vi "纳清电导率电极校准.vi"() -> ()   [LabVIEW 2016, in "斯坦道多参数.lvlib"]
uses:
  <vilib>/Utility/miscctls.llb/LVPointTypeDef.ctl
  <vilib>/Analysis/NI_AALBase.lvlib
panel:
  out "滤波设定":sgl
  out "第二点信号值":dbl
  out "第一点信号值":dbl
  out "盐度":dbl caption="盐度测量值" format="%#.2f"
  out "当前量程":u16
  out "报警信息":string
  out "通讯状态":string
  out "第二点校准值":dbl
  out "第一点校准值":dbl
  in  "校准停止":bool
  in  "校准启动":bool
  in  "校准模式":u16(ring) items=["单点校准"]
  out "最小值":sgl format="%#.2f"
  out "最大值":sgl format="%#.2f"
  out "波形图表":dbl(graph) caption="历史曲线"
  out "mean":dbl caption="均值" format="%#.2f"
  out "standard deviation":dbl caption="标准差" format="%#.2f"
  out "变异系数":dbl format="%#.6f"
  out "测量值":sgl format="%#.2f"
  out "提示":string
  out "标液1":sgl
  out "原始光强数值":sgl caption="信号值" format="%#.6f"
  out "温度":dbl format="%#.2f"
  # "电导率电极设定"
  # "℃"
  # "μS/cm"
  # "ppt"
  # "电阻"
  # "请选择校准模式:"
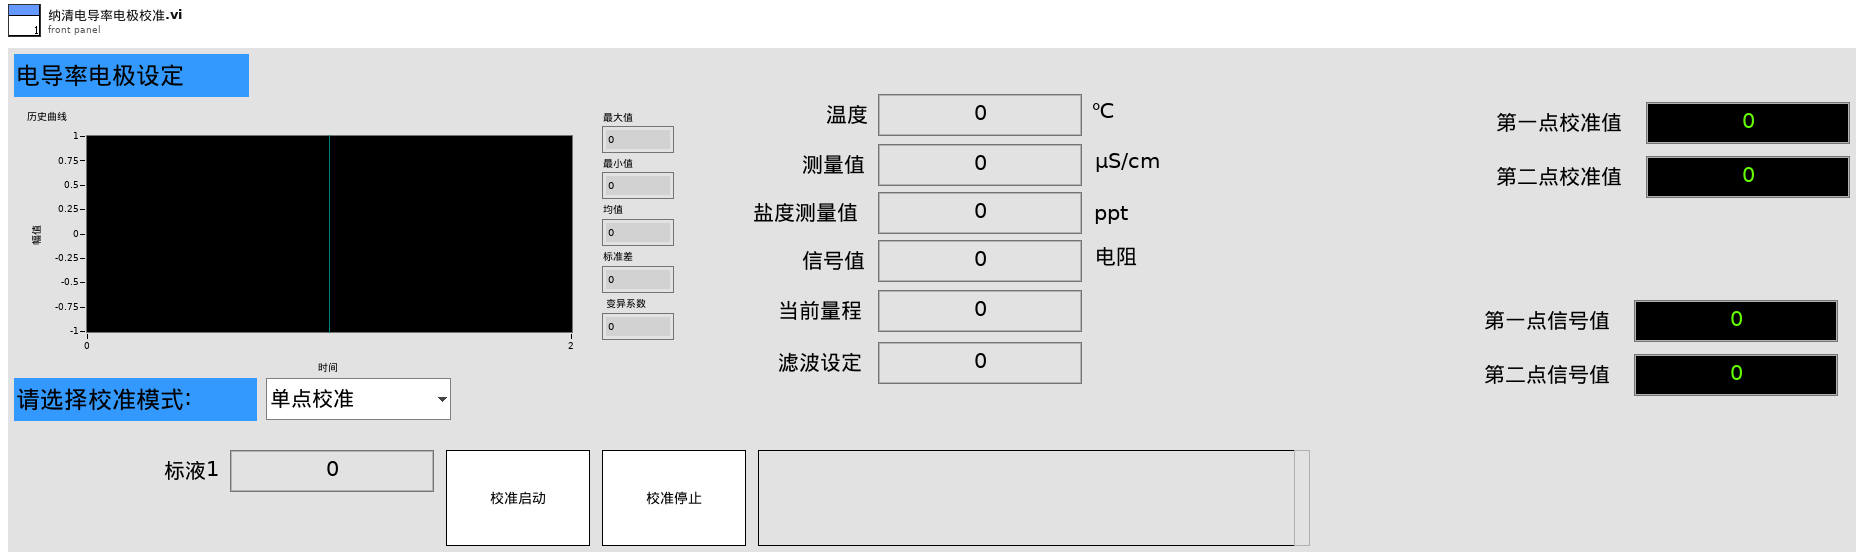
[diagram p1: front panel]
types:
  T1 = enum16{"pH", "DO", "Cond", "Turb", "ORP", "叶绿素a", "藻密度"}
  T2 = typedef "LVPointTypeDef.ctl" = cluster{"Horizontal":i16, "Vertical":i16}
  T3 = cluster{"报警码":u16, "电导率数据（uS/cm）":sgl, "0x0003 NC":sgl, "温度数据":sgl, "电导率原始信号电阻":sgl, "当前量程":u16, "温度补偿系数":sgl, "0X0009_NC":string, "产品名称":string, "序列号":string, "硬件版本":string, "软件版本":string, "通讯地址":u16, "波特率":u16, "设备类型":u16, "0X0026_NC":string, "第一点原始数据":sgl, "第一点校准数据":sgl, "0X0035_NC":sgl, "0X0037_NC":sgl, "探头校准命令":u16, "温度校准参数":sgl, "温度校准命令":u16}
  T4 = cluster{"温度测量值":sgl, "测量值":sgl, "温度偏移修正值":sgl, "信号值":sgl}
  T5 = cluster{"pH":u32, "DO":u32, "Cond":u32, "Turb":u32, "叶绿素a":u32, "藻密度":u32, "ORP":u32}
  T6 = enum8{"Enabled", "Disabled", "Disabled and Grayed Out"}
  T7 = cluster{"ph":bool, "DO":bool, "Cond":bool, "Turb":bool, "叶绿素a":bool, "藻密度":bool, "ORP":bool}
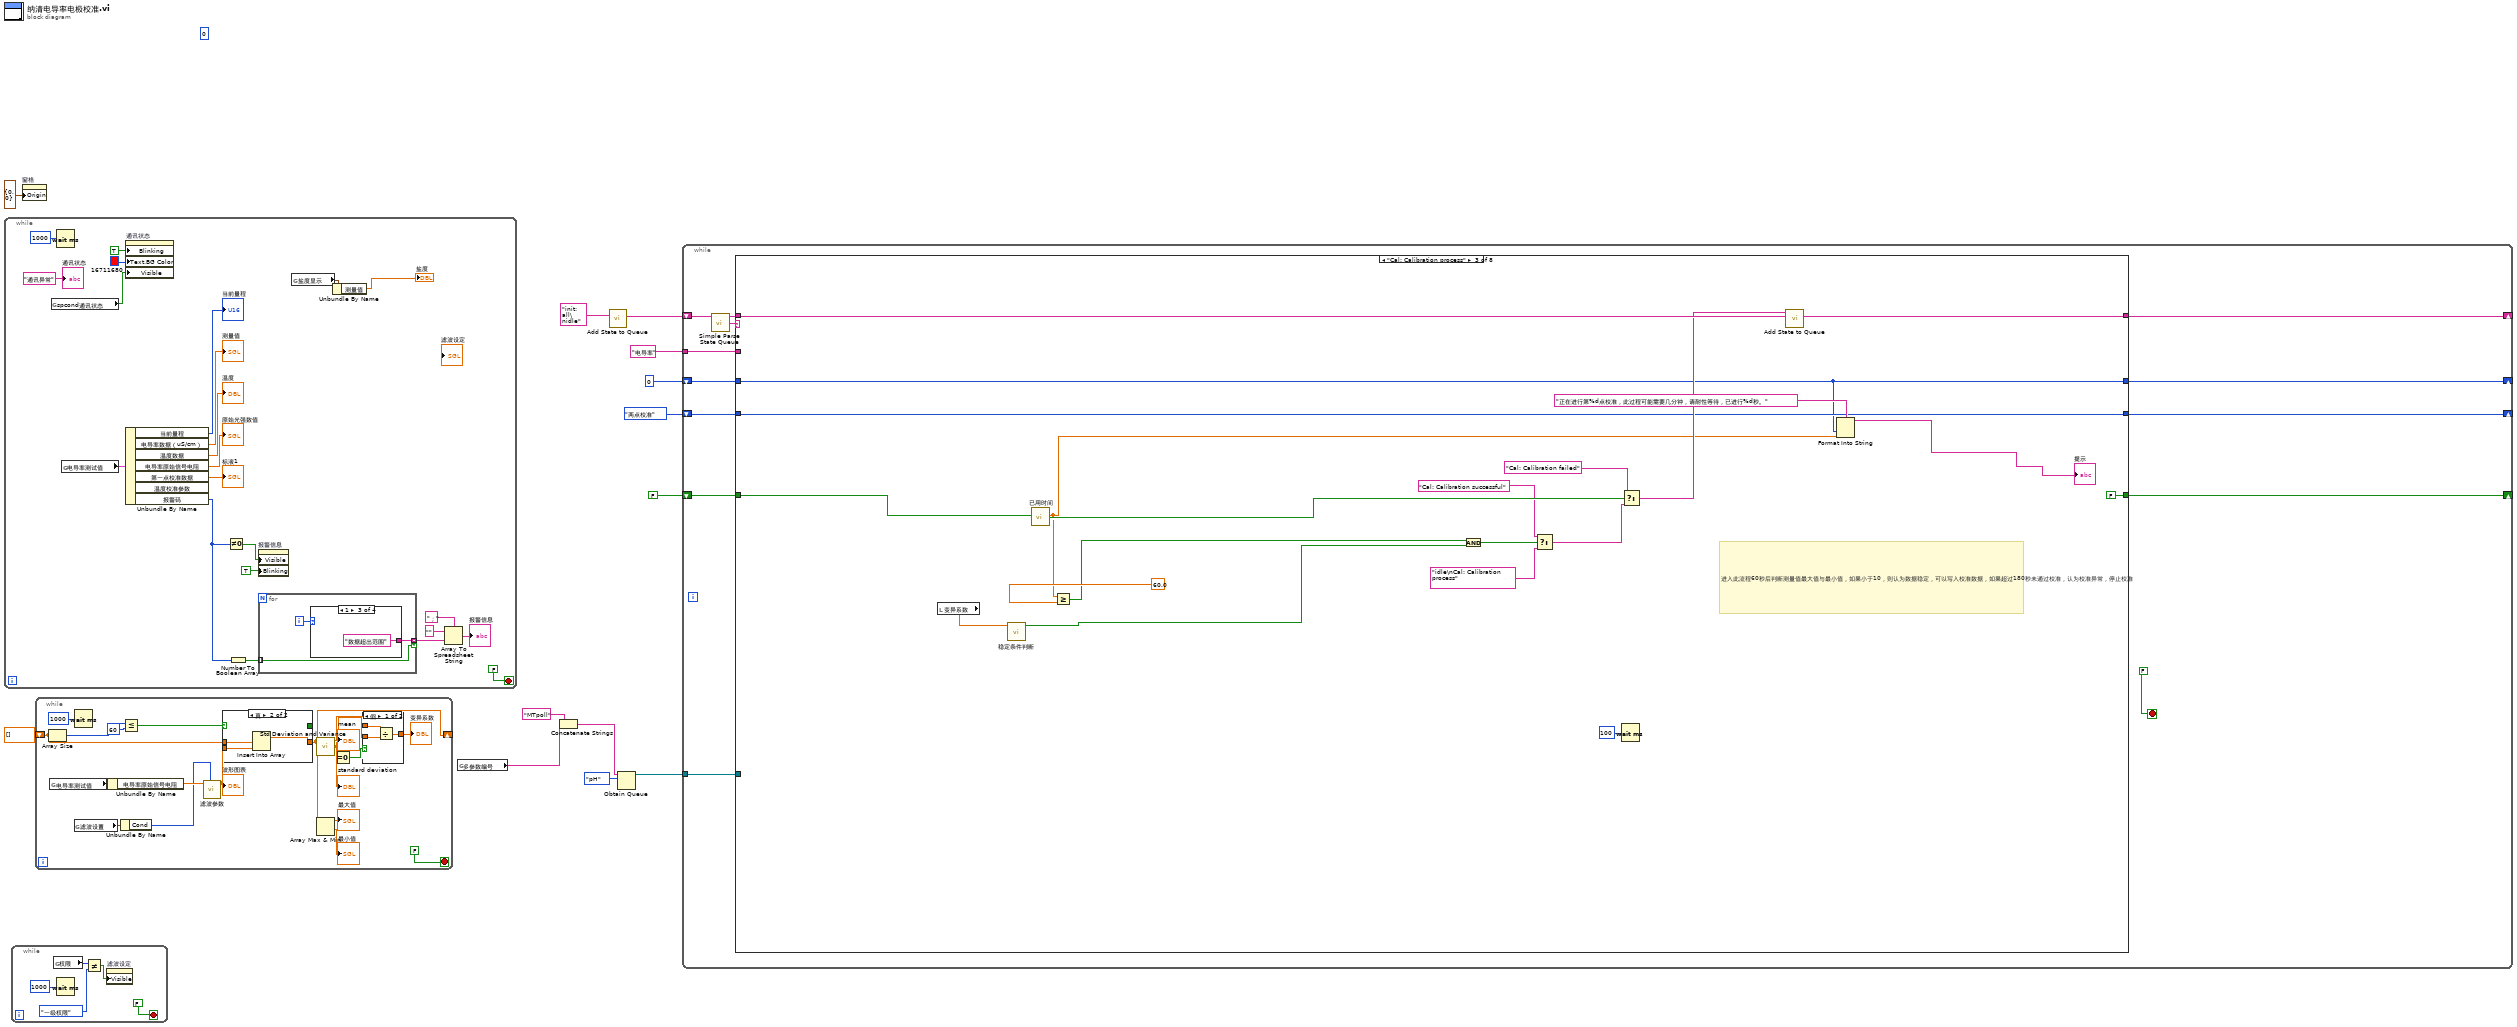
[diagram p0: block diagram]
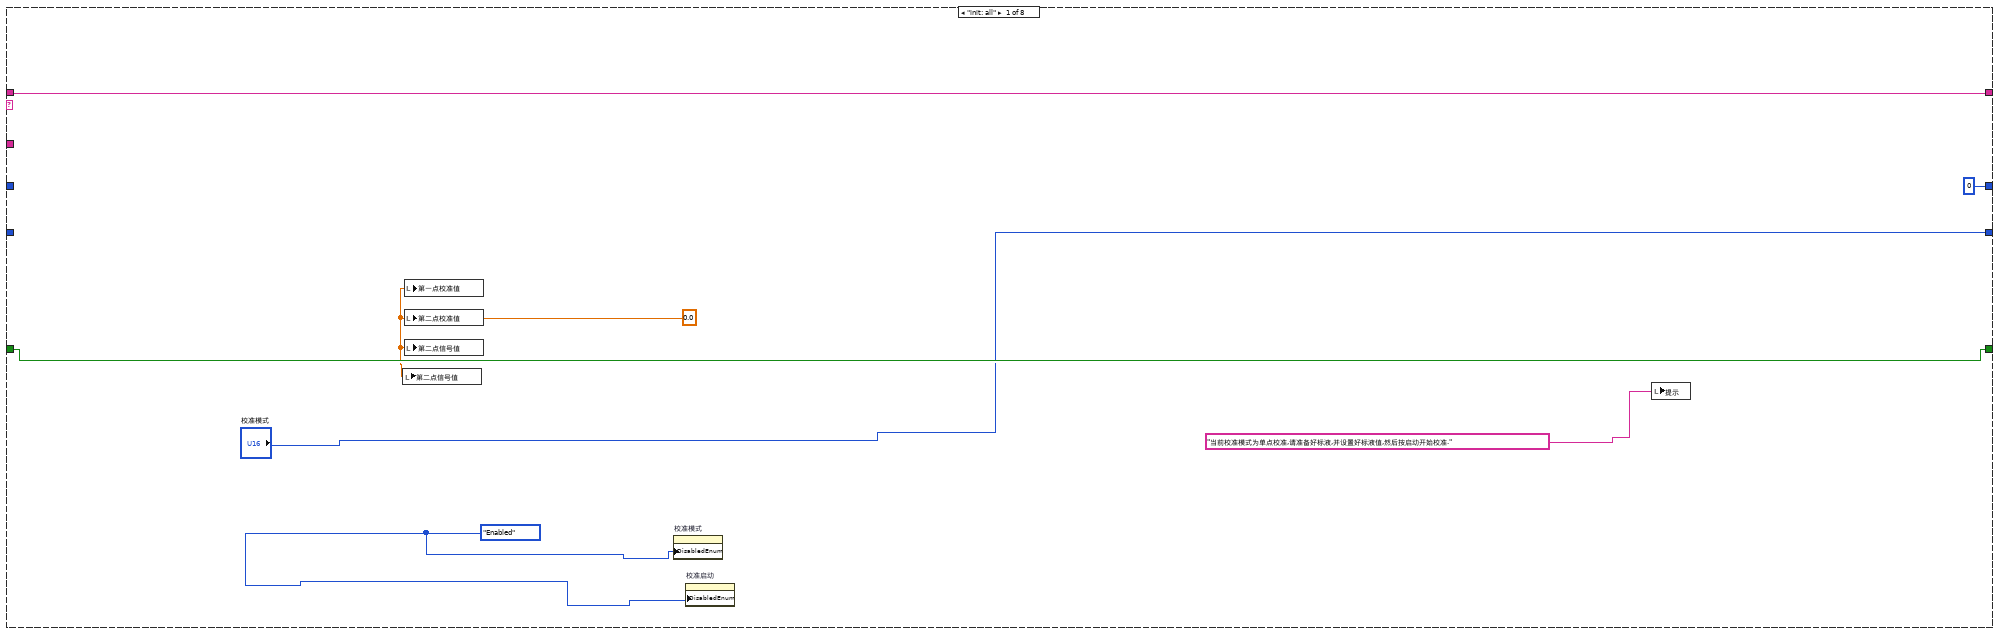
[diagram p2: hidden frame]
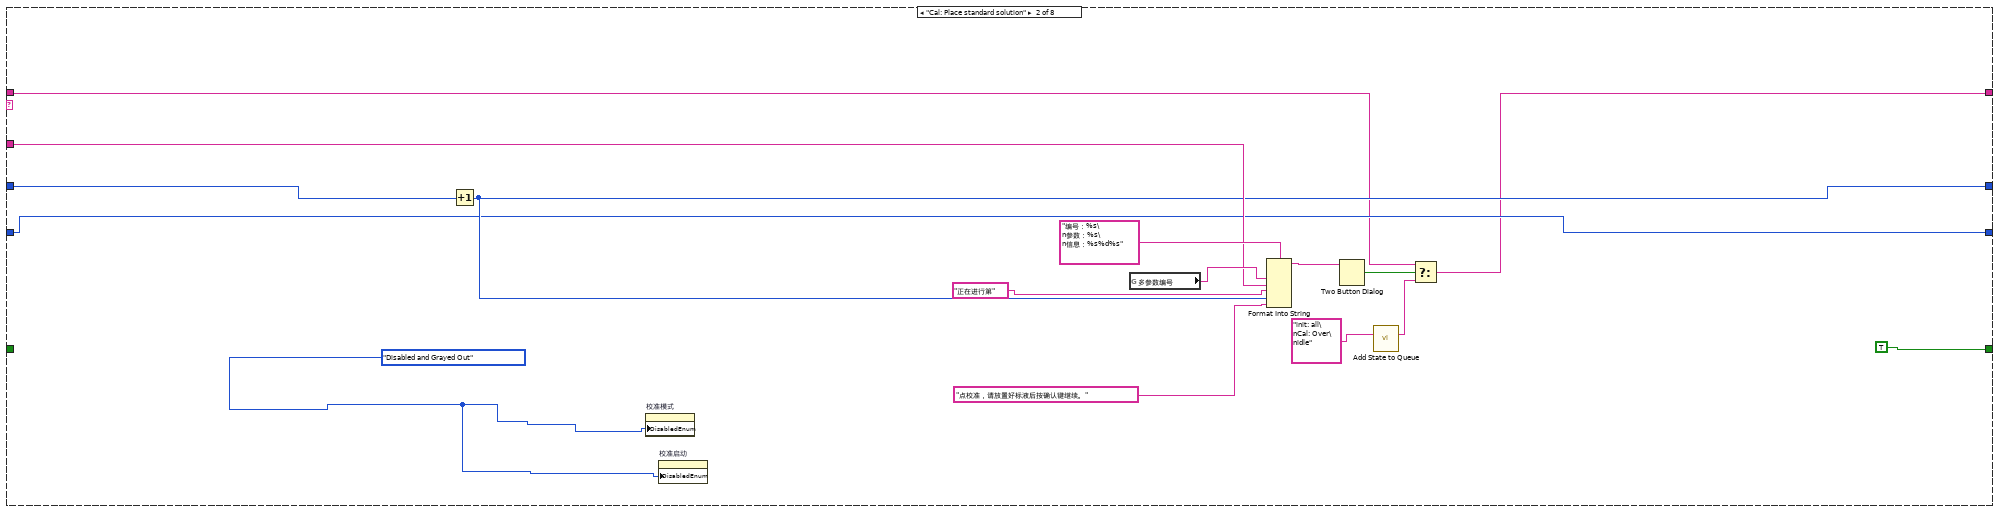
[diagram p3: hidden frame]
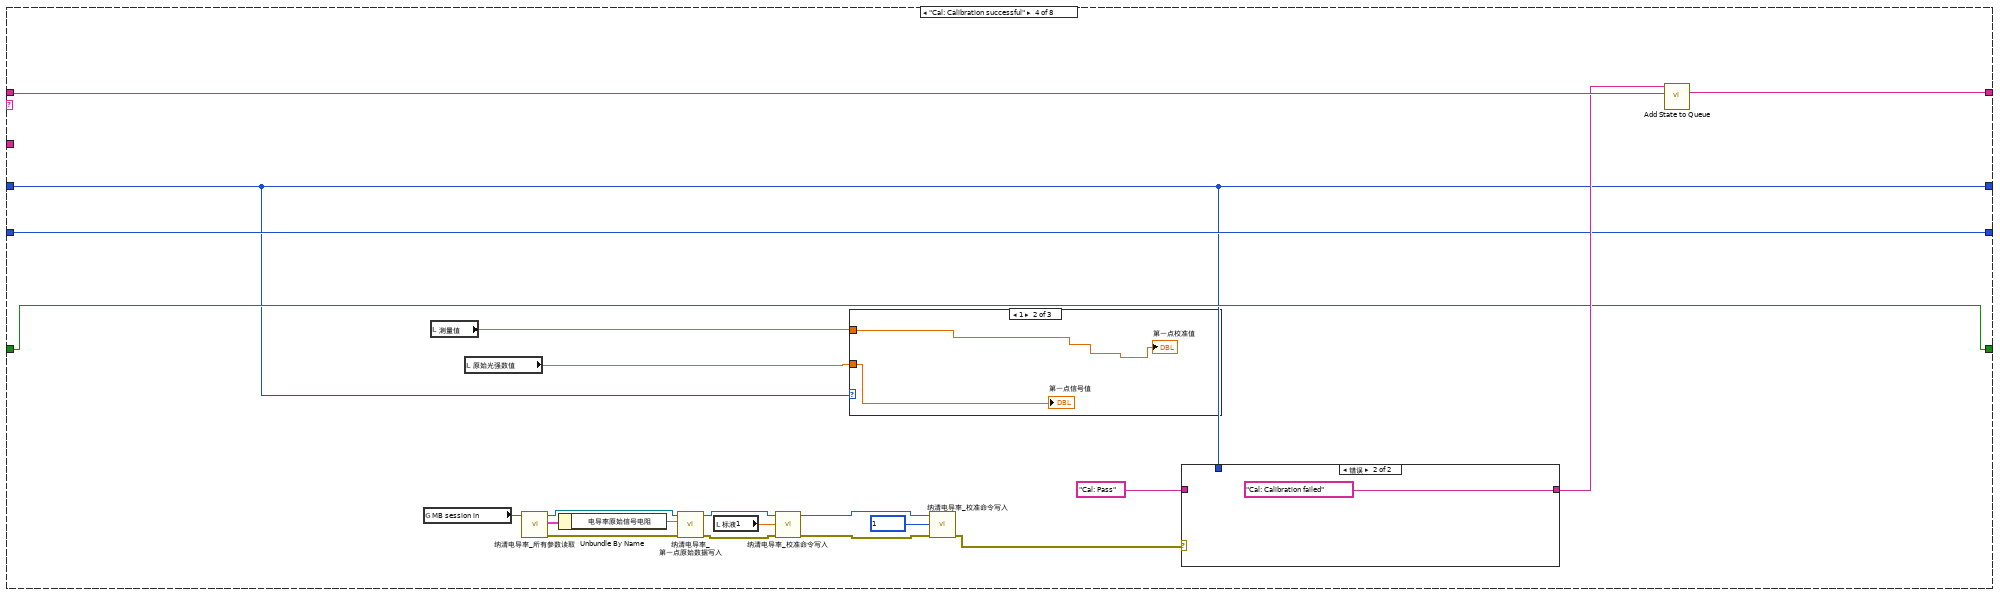
[diagram p4: hidden frame]
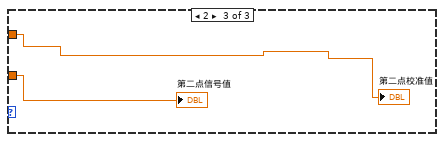
[diagram p6: hidden frame]
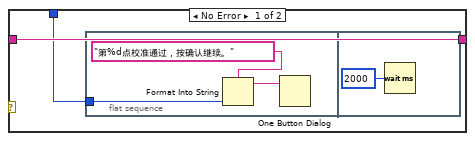
[diagram p7: hidden frame]
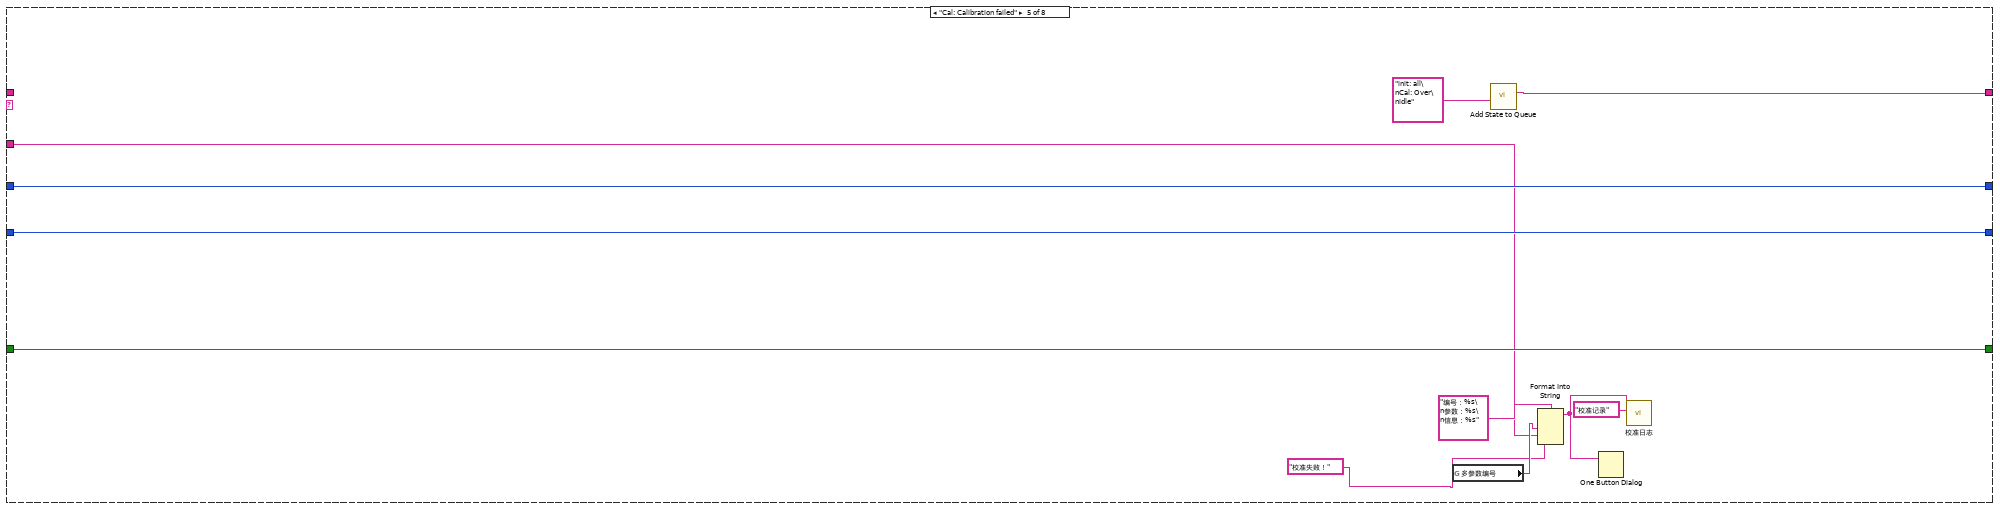
[diagram p8: hidden frame]
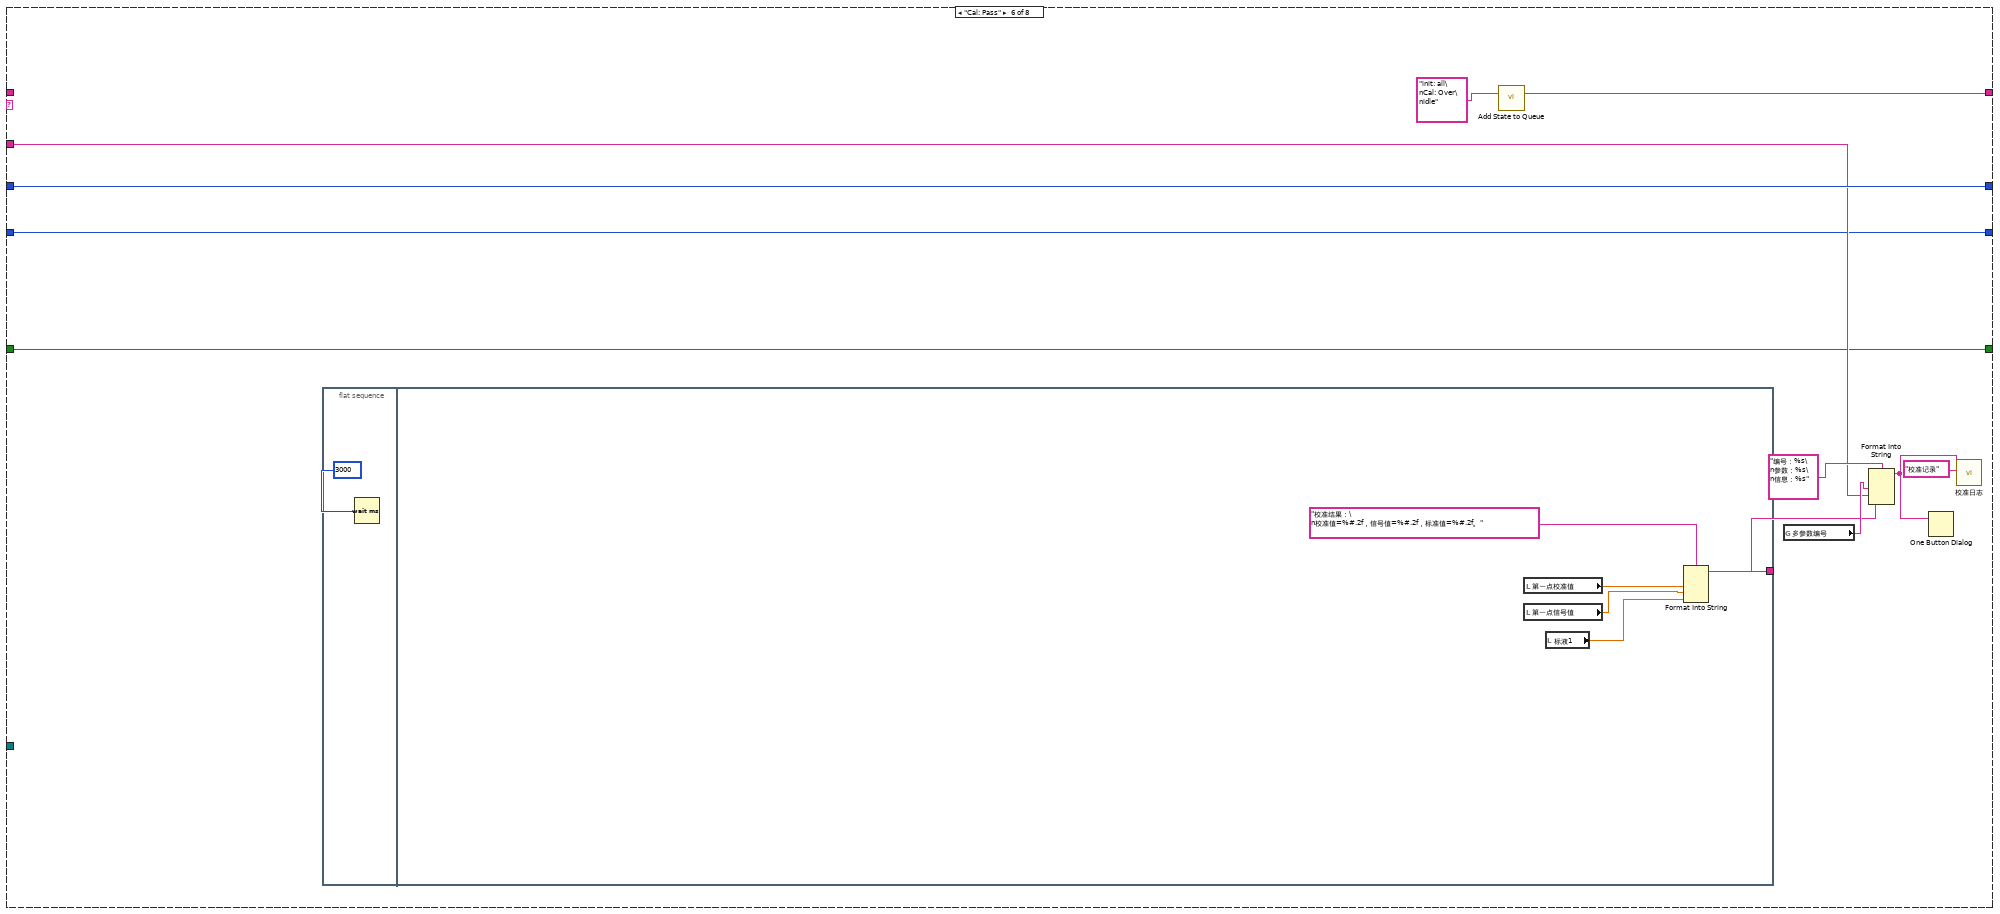
[diagram p9: hidden frame]
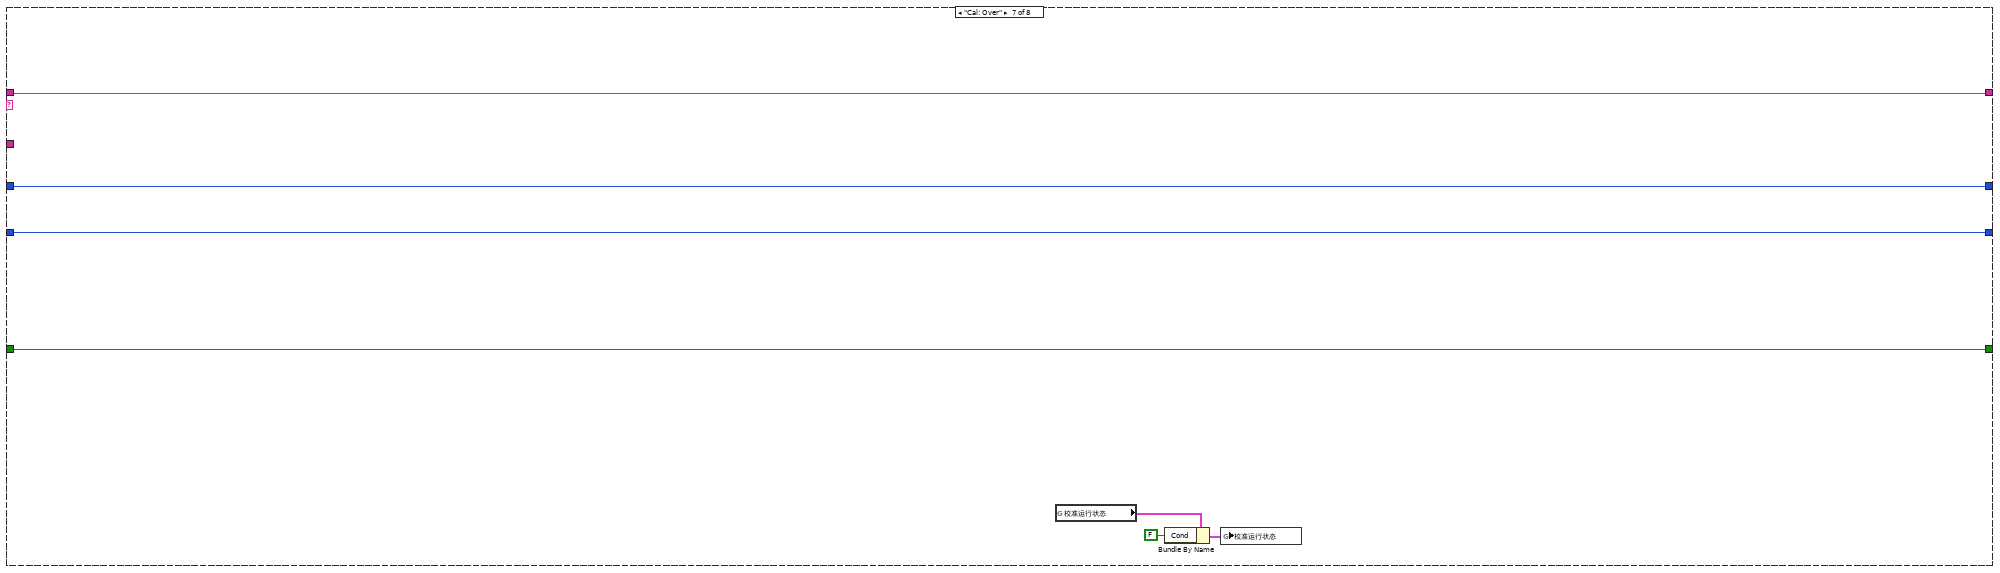
[diagram p10: hidden frame]
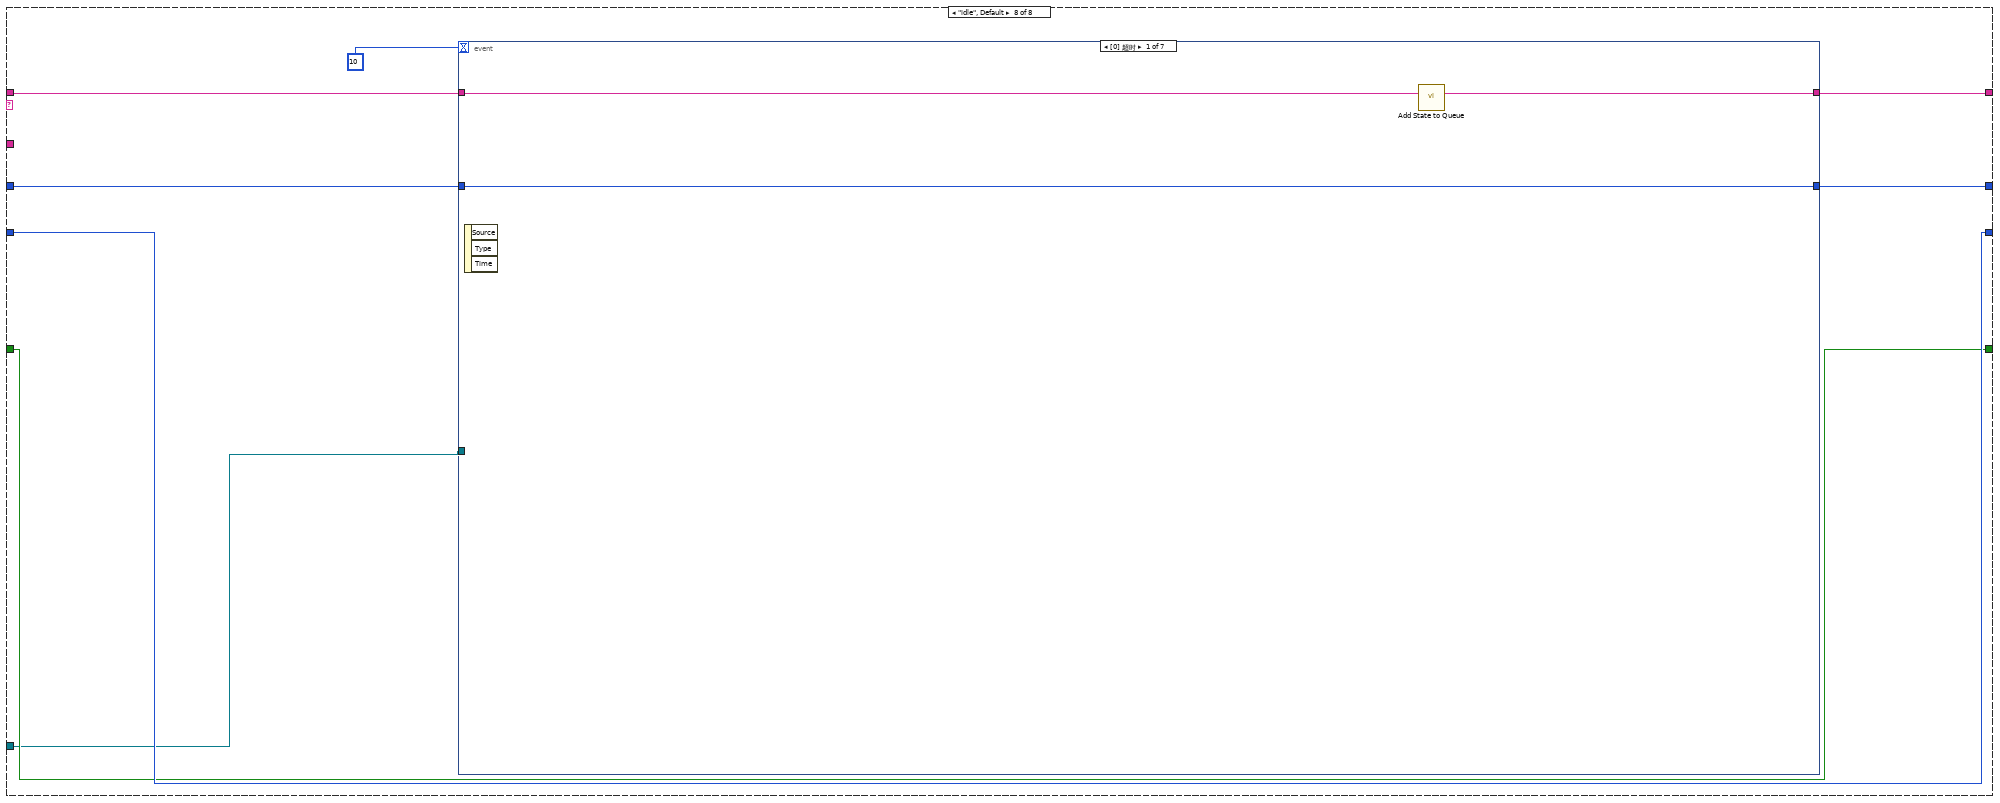
[diagram p11: hidden frame]
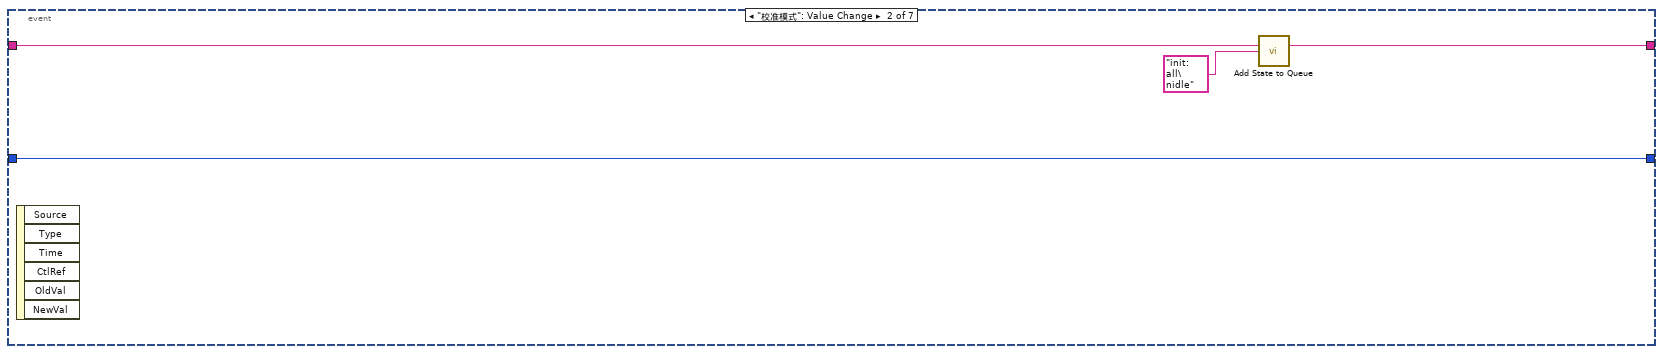
[diagram p12: hidden frame]
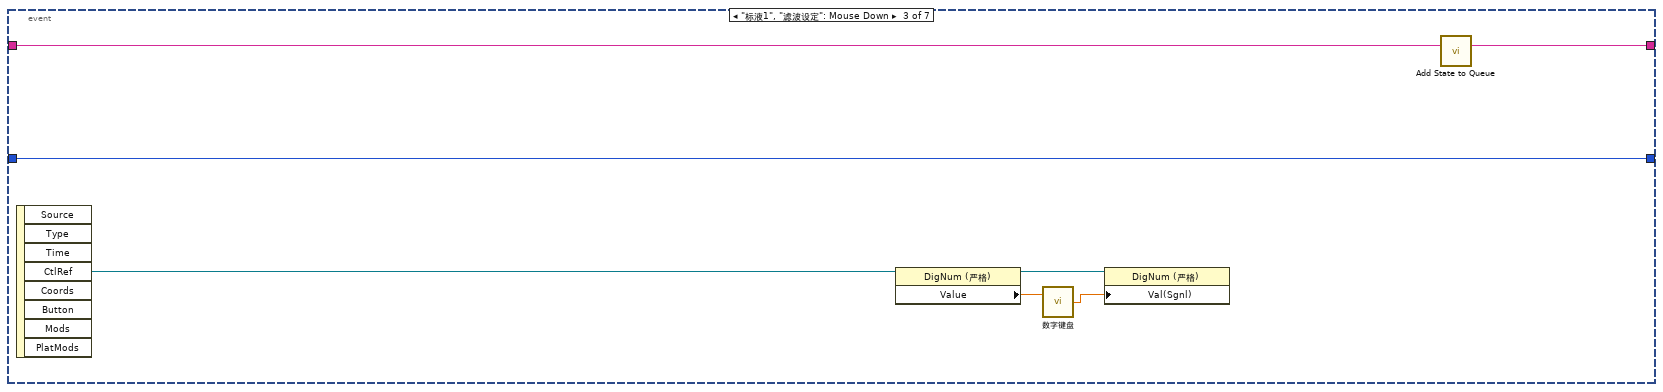
[diagram p13: hidden frame]
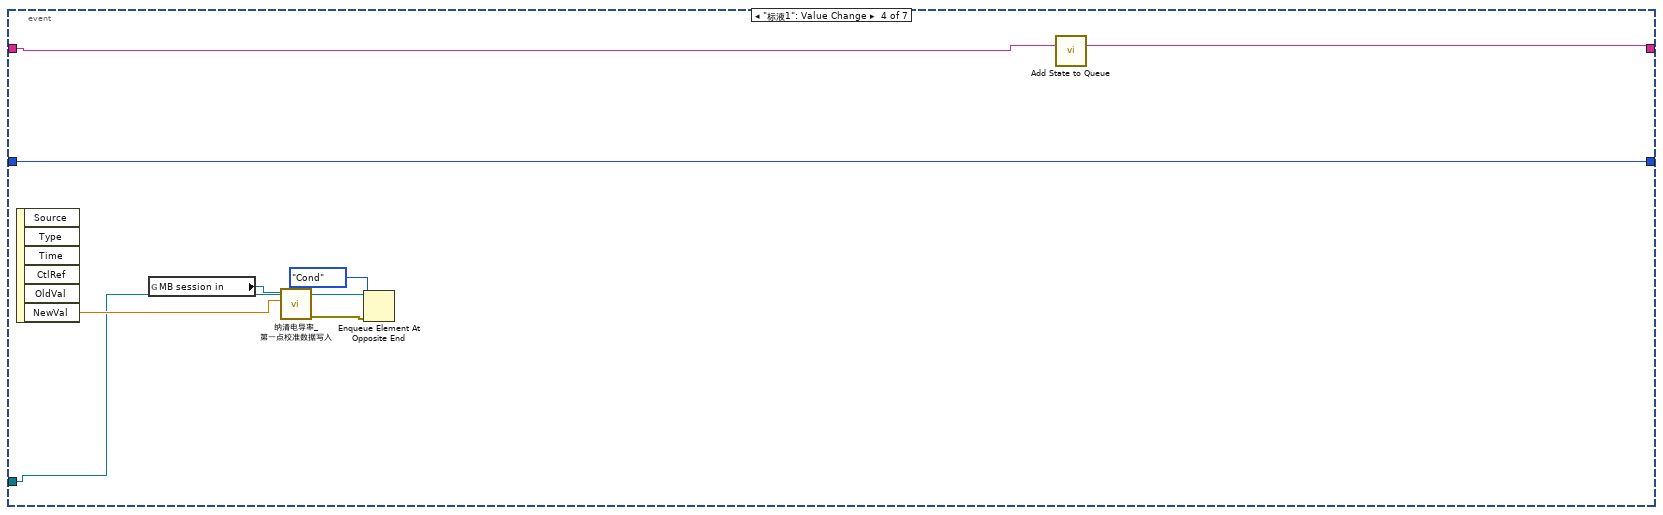
[diagram p14: hidden frame]
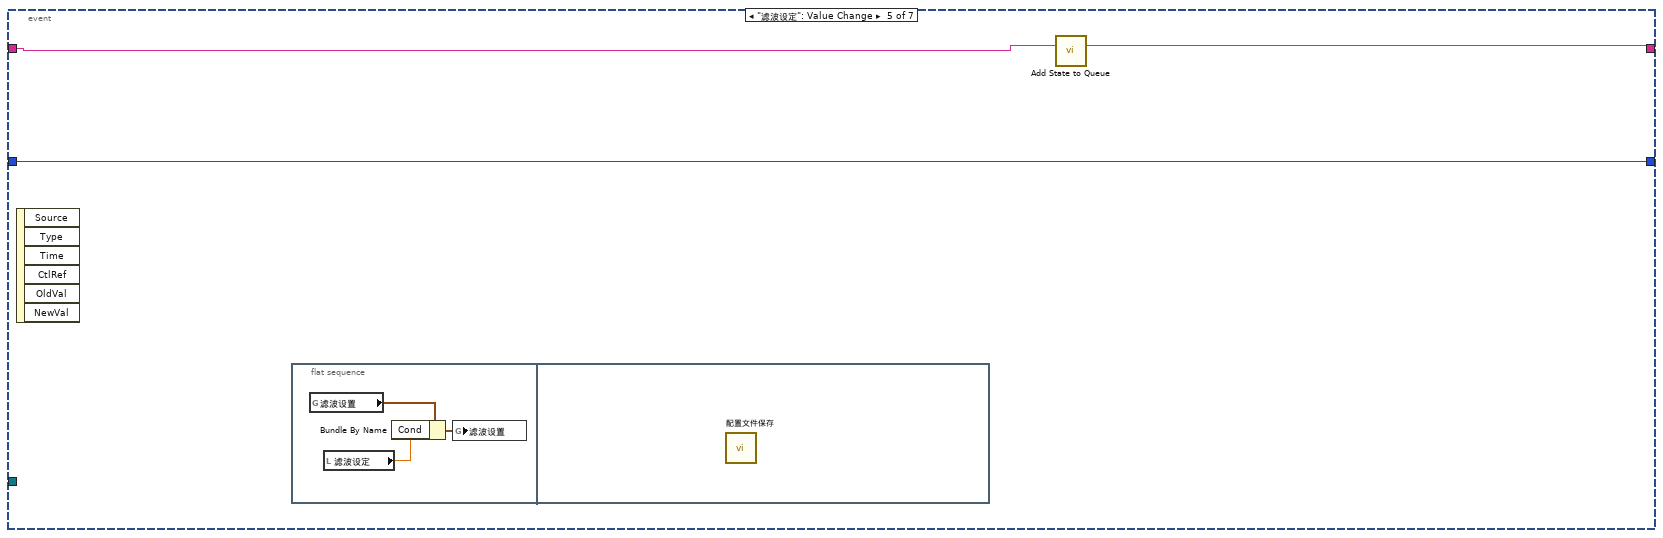
[diagram p15: hidden frame]
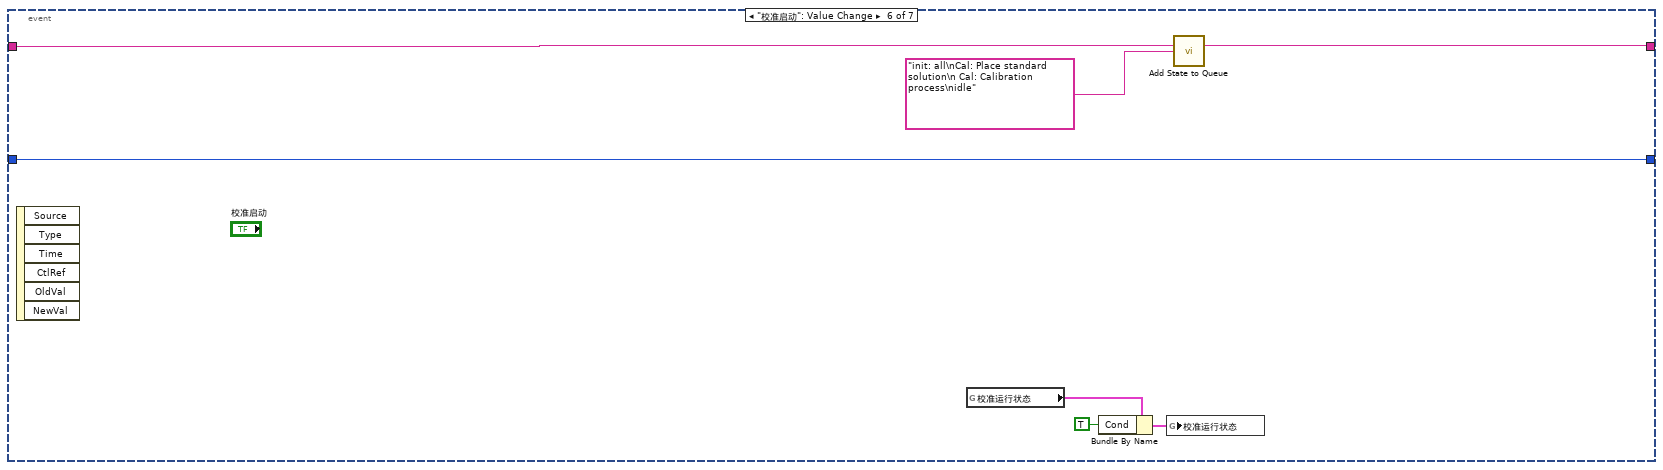
[diagram p16: hidden frame]
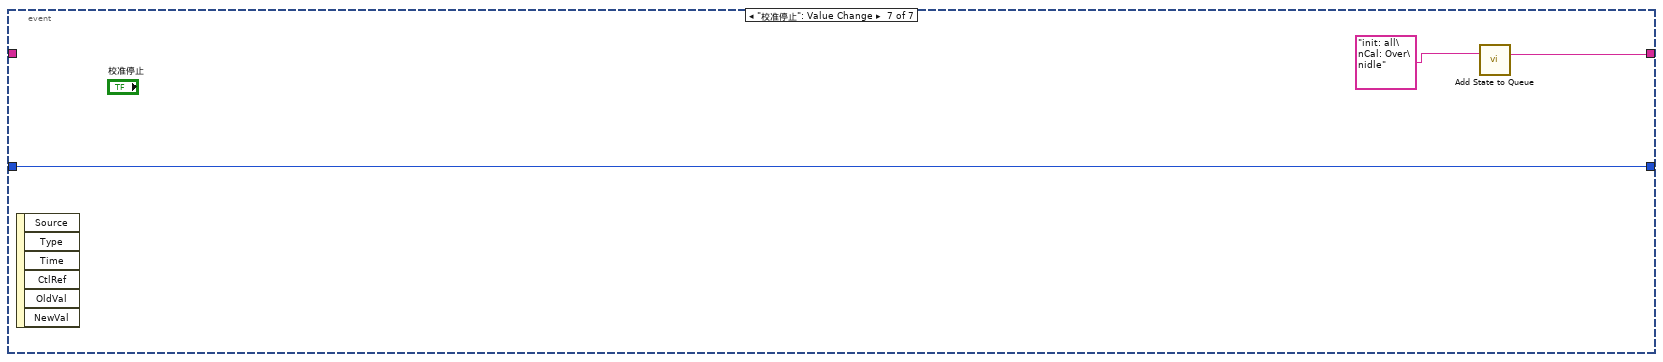
[diagram p17: hidden frame]
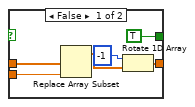
[diagram p19: hidden frame]
diagram:
  (unwired) 0
  n1 = while {
    stop <- FALSE stop-if-true
    n2 = global read "多参数全局变量.vi" "spcond通讯状态"() -> (w25:bool)
    n3 = Wait (ms)(milliseconds to wait=u32 1000 ("等待时间（毫秒）")) -> ()  [unwired: 1 out]
    n4 = global read "纳清过程全局变量.vi" "电导率测试值"() -> (w33:T3)
    n5 = property on="通讯状态" class="Str"("Blinking"=TRUE ("闪烁"), "Text.BG Color"=u32 16711680, "Visible"=w25) -> ()  [unwired: 2 in, 2 out]
    n6 = Unbundle By Name(w33) -> ("当前量程"=→"当前量程":u16, "电导率数据（uS/cm）"=→"测量值":sgl, "温度数据"=→"温度":sgl, "电导率原始信号电阻"=→"原始光强数值":sgl, "第一点校准数据"=→"标液1":sgl, "报警码"=w19:u16)  [unwired: 1 out]
    n7 = Not Equal To 0?(x=w19) -> (x != 0?=w18:bool)
    n8 = Number To Boolean Array(number=w19) -> (Boolean array=w24:bool[])
    n9 = property on="报警信息" class="Str"("Visible"=w18, "Blinking"=TRUE ("闪烁")) -> ()  [unwired: 2 in, 2 out]
    n10 = for {
      tunnel: w24 -> [w36] mode=indexing
      tunnel: [w37] -> w23 mode=indexing if=w36
      i -> [w38]
      n11 = case shown="1" w38 {
        tunnel: [_ "温度超出范围" "数据超出范围" "温度传感器故障"] -> w37
        frame Default {
        }
        frame 0 {
        }
        frame 1 {
        }
        frame 8 {
        }
      }
    }
    n12 = global read "多参数全局变量.vi" "盐度显示"() -> (w14:T4)
    n13 = Unbundle By Name(w14) -> ("测量值"=→"盐度":sgl)
    n14 = Array To Spreadsheet String(delimiter (Tab)="；" ("分隔符(Tab)"), array=w23, 3:"" ("格式字符串")) -> (spreadsheet string=→"报警信息":string)
    "通讯状态" <- "通讯异常" ("当前串口")
  }
  n15 = while {
    stop <- FALSE stop-if-true
    n16 = global read "多参数全局变量.vi" "权限"() -> (w45:enum16{"一级权限", "二级权限", "三级权限"})
    n17 = Wait (ms)(milliseconds to wait=u32 1000 ("等待时间（毫秒）")) -> ()  [unwired: 1 out]
    n18 = Not Equal?(x=w45, y=enum16{"一级权限", "二级权限", "三级权限"}."一级权限") -> (x != y?=w42:bool)
    n19 = property on="滤波设定" class="DigNum (严格)"("Visible"=w42) -> ()  [unwired: 2 in, 2 out]
  }
  n20 = property on="窗格" class="Pane"("Origin"=T2 {"Horizontal"=0, "Vertical"=0} ("原点")) -> ()  [unwired: 2 in, 2 out]
  n21 = while {
    shift-right: [w54] -> _
    shift-left: sgl[] [] -> [w60]
    stop <- FALSE stop-if-true
    n22 = Array Size(array=w60) -> (size(s)=w62:i32)
    n23 = global read "纳清过程全局变量.vi" "电导率测试值"() -> (w51:T3)
    n24 = global read "断电保存变量.vi" "滤波设置"() -> (w48:T5)
    n25 = Wait (ms)(milliseconds to wait=u32 1000 ("等待时间（毫秒）")) -> ()  [unwired: 1 out]
    n26 = Unbundle By Name(w51) -> ("电导率原始信号电阻"=w50:sgl)
    n27 = Unbundle By Name(w48) -> ("Cond"=w47:u32)
    n28 = Less Or Equal?(x=w62, y=60) -> (x <= y?=w61:bool)
    n29 = call "滤波参数.vi"("滤波次数"=w47, "x"=w50) -> ("mode"=w49:dbl)  [unwired: 9 in]
    "波形图表" <- w49
    n30 = case shown="真" w61 {
      tunnel: w60 -> [w73 w76]
      tunnel: w49 -> [w71 w75]
      tunnel: [w69 w74] -> w54
      tunnel: [TRUE _] -> _
      frame False {
        n31 = Replace Array Subset(array=w73, new element=w71) -> (w72:sgl[])  [unwired: 1 in]
        n32 = Rotate 1D Array(1:w72, 2:-1 ("n")) -> (0:w69:sgl[])
      }
      frame True {
        n33 = Insert Into Array(array=w76, new element=w75) -> (w74:sgl[])  [unwired: 1 in]
      }
    }
    n34 = call <vilib>:"Std Deviation and Variance.vi"("X"=w54) -> ("mean"=w58:dbl, "standard deviation"=w57:dbl)  [unwired: 1 in, 1 out]
    "mean" <- w58
    "standard deviation" <- w57
    n35 = Array Max & Min(array=w54) -> (max value=→"最大值":sgl, min value=→"最小值":sgl)  [unwired: 2 out]
    n36 = Equal To 0?(x=w58) -> (x = 0?=w59:bool)
    n37 = case shown="假" w59 {
      tunnel: w57 -> [w67 _]
      tunnel: [w66 _] -> w56
      tunnel: w58 -> [w65 _]
      frame False {
        n38 = Divide(x=w67, y=w65) -> (x/y=w66:dbl)
      }
      frame True {
      }
    }
    "变异系数" <- w56
  }
  n39 = global read "多参数全局变量.vi" "多参数编号"() -> (w2:string)
  n40 = Concatenate Strings("MTpoll" ("名称（未命名）"), w2) -> (w4:string)
  n41 = call "Add State to Queue.vi"("State(s) In (\"\")"="init: all\nidle" ("State(s) In (\"\")")) -> ("States Out"=w10:string)  [unwired: 14 in]
  n42 = Obtain Queue(name (unnamed)=w4, element data type=T1."pH" ("枚举")) -> (queue out=w1:refnum<queue>)  [unwired: 3 in, 2 out]
  n43 = while {
    shift-right: [w85] -> _
    shift-left: w10 -> [w89]
    shift-right: [w82] -> _
    shift-left: 0 -> [w84]
    tunnel: "电导率" ("State(s) In (\"\")") -> [w83]
    shift-right: [w80] -> _
    shift-left: enum16{"两点校准", "单点校准"}."两点校准" ("校准模式") -> [w81]
    shift-right: [w78] -> _
    shift-left: FALSE -> [w79]
    tunnel: w1 -> [w77]
    stop <- FALSE stop-if-true
    n44 = call "Simple Parse State Queue.vi"("State Queue"=w89) -> ("Remain States"=w86:string, "Next State"=w87:string)  [unwired: 13 in]
    n45 = case shown="\"Cal: Calibration process\"" w87 {
      tunnel: w86 -> [w96 w99 w132 w153 _ _ w200 w208]
      tunnel: [w96 w98 w131 w152 w173 w177 w200 w207] -> w85
      tunnel: w84 -> [_ w108 w117 w135 w176 w187 w199 w205]
      tunnel: w83 -> [_ w109 _ _ w166 w183 _ _]
      tunnel: [0 w106 w117 w135 w176 w187 w199 w206] -> w82
      tunnel: w81 -> [_ w105 w118 w147 w175 w179 w198 w204]
      tunnel: ["校准模式" w105 w118 w147 w175 w179 w198 w204] -> w80
      tunnel: w79 -> [w93 _ w120 w148 w174 w182 w197 w202]
      tunnel: [w93 TRUE FALSE w148 w174 w182 w197 w202] -> w78
      tunnel: w77 -> [_ _ _ _ _ _ _ w201]
      frame "init: all" {
        w90 = T6."Enabled" ("禁用")
        w92 = 0.0 ("第一点校准值")
        n46 = local write "第二点信号值"(w92) -> ()
        n47 = local write "第一点校准值"(w92) -> ()
        n48 = local write "第二点校准值"(w92) -> ()
        n49 = local write "第二点信号值"(w92) -> ()
        n50 = property on="校准模式" class="Ring (严格)"("DisabledEnum"=w90) -> ()  [unwired: 2 in, 2 out]
        n51 = property on="校准启动" class="Bool"("DisabledEnum"=w90) -> ()  [unwired: 2 in, 2 out]
        n52 = local write "提示"("当前校准模式为单点校准,请准备好标液,并设置好标液值,然后按启动开始校准." ("提示")) -> ()
      }
      frame "Cal: Place standard solution" {
        w97 = T6."Disabled and Grayed Out" ("禁用")
        n53 = Increment(x=w108) -> (x+1=w106:i32)
        n54 = property on="校准模式" class="Ring (严格)"("DisabledEnum"=w97) -> ()  [unwired: 2 in, 2 out]
        n55 = property on="校准启动" class="Bool"("DisabledEnum"=w97) -> ()  [unwired: 2 in, 2 out]
        n56 = global read "多参数全局变量.vi" "多参数编号"() -> (w111:string)
        n57 = Format Into String(format string="编号：%s\n参数：%s\n信息：%s%d%s" ("格式字符串"), w111, w109, "正在进行第" ("消息"), w106, "点校准，请放置好标液后按确认键继续。" ("消息")) -> (resulting string=w103:string)  [unwired: 2 in, 1 out]
        n58 = Two Button Dialog(message=w103) -> (T button?=w102:bool)  [unwired: 2 in]
        n59 = call "Add State to Queue.vi"("State(s) In (\"\")"="init: all\nCal: Over\nidle" ("State(s) In (\"\")")) -> ("States Out"=w100:string)  [unwired: 14 in]
        n60 = Select(t=w99, s=w102, f=w100) -> (s? t:f=w98:string)
      }
      frame "Cal: Calibration process" {
        # "进入此流程60秒后判断测量值最大值与最小值，如果小于10，则认为数据稳定，可以写入校准数据，如果超过180秒未通过校准，认为校准异常，停止校准"
        n61 = local read "变异系数"() -> (w114:dbl)
        n62 = call "稳定条件判断.vi"("变异系数"=w114) -> ("布尔"=w113:bool)  [unwired: 10 in]
        n63 = call "已用时间"("Reset"=w120) -> ("Elapsed Time (s)"=w116:dbl, "Time has Elapsed"=w133:bool)  [unwired: 11 in, 6 out]
        n64 = Greater Or Equal?(x=w116, y=60.0) -> (x >= y?=w128:bool)
        n65 = And(x=w128, y=w113) -> (x .and. y?=w125:bool)
        n66 = Select(t="Cal: Calibration successful" ("State(s) In (\"\")"), s=w125, f="idle\nCal: Calibration process" ("State(s) In (\"\")")) -> (s? t:f=w124:string)
        n67 = Wait (ms)(milliseconds to wait=u32 100 ("等待时间（毫秒）")) -> ()  [unwired: 1 out]
        n68 = Select(t="Cal: Calibration failed" ("State(s) In (\"\")"), s=w133, f=w124) -> (s? t:f=w123:string)
        n69 = call "Add State to Queue.vi"("State(s) In Front (\"\")"=w123, "State(s) In (\"\")"=w132) -> ("States Out"=w131:string)  [unwired: 13 in]
        n70 = Format Into String(format string="正在进行第%d点校准，此过程可能需要几分钟，请耐性等待，已进行%d秒。" ("格式字符串"), w117, w116) -> (resulting string=→"提示":string)  [unwired: 2 in, 1 out]
      }
      frame "Cal: Calibration successful" {
        n71 = global read "多参数全局变量.vi" "MB session in"() -> (w139:refnum<class "MB_Master.lvclass">)
        n72 = local read "测量值"() -> (w149:sgl)
        n73 = local read "原始光强数值"() -> (w150:sgl)
        n74 = call "纳清电导率_所有参数读取.vi"("MB session in"=w139) -> ("error out"=w137:errorcluster, "输出值"=w140:T3, "MB session out"=w138:refnum<class "MB_Master.lvclass">)  [unwired: 8 in]
        n75 = Unbundle By Name(w140) -> ("电导率原始信号电阻"=w141:sgl)
        n76 = call "纳清电导率_第一点原始数据写入.vi"("error in (no error)"=w137, "数值"=w141, "MB session in"=w138) -> ("error out"=w142:errorcluster, "MB session out"=w143:refnum<class "MB_Master.lvclass">)  [unwired: 7 in]
        n77 = local read "标液1"() -> (w146:sgl)
        n78 = call "纳清电导率_校准命令写入.vi"("error in (no error)"=w142, "数值"=w146, "MB session in"=w143) -> ("error out"=w144:errorcluster, "MB session out"=w145:refnum<class "MB_Master.lvclass">)  [unwired: 7 in]
        n79 = case shown="1" w135 {
          tunnel: w150 -> [_ w156 w158]
          tunnel: w149 -> [_ w155 w157]
          frame 0, Default {
          }
          frame 1 {
            "第一点信号值" <- w156
            "第一点校准值" <- w155
          }
          frame 2 {
            "第二点信号值" <- w158
            "第二点校准值" <- w157
          }
        }
        n80 = call "纳清电导率_校准命令写入.vi"("error in (no error)"=w144, "数值"=u16 1 ("starting address"), "MB session in"=w145) -> ("error out"=w134:errorcluster)  [unwired: 7 in, 1 out]
        n81 = case shown="错误" w134 {
          tunnel: "Cal: Pass" ("State(s) In (\"\")") -> [w160 _]
          tunnel: [w160 "Cal: Calibration failed" ("State(s) In (\"\")")] -> w151
          tunnel: w135 -> [w159 _]
          frame No Error {
            n82 = flat-sequence {
              tunnel: w159 -> [w161]
              frame #0 {
                n83 = Format Into String(format string="第%d点校准通过，按确认继续。" ("格式字符串"), w161) -> (resulting string=w163:string)  [unwired: 2 in, 1 out]
                n84 = One Button Dialog(message=w163) -> ()  [unwired: 1 in, 1 out]
              }
              frame #1 {
                n85 = Wait (ms)(milliseconds to wait=u32 2000 ("等待时间（毫秒）")) -> ()  [unwired: 1 out]
              }
            }
          }
          frame Error {
          }
        }
        n86 = call "Add State to Queue.vi"("State(s) In Front (\"\")"=w151, "State(s) In (\"\")"=w153) -> ("States Out"=w152:string)  [unwired: 13 in]
      }
      frame "Cal: Calibration failed" {
        n87 = global read "多参数全局变量.vi" "多参数编号"() -> (w169:string)
        n88 = call "Add State to Queue.vi"("State(s) In (\"\")"="init: all\nCal: Over\nidle" ("State(s) In (\"\")")) -> ("States Out"=w173:string)  [unwired: 14 in]
        n89 = Format Into String(format string="编号：%s\n参数：%s\n信息：%s" ("格式字符串"), w169, w166, "校准失败！" ("消息")) -> (resulting string=w168:string)  [unwired: 2 in, 1 out]
        n90 = One Button Dialog(message=w168) -> ()  [unwired: 1 in, 1 out]
        n91 = call "校准日志.vi"("table"="校准记录", "日志信息"=w168) -> ()  [unwired: 9 in, 1 out]
      }
      frame "Cal: Pass" {
        n92 = flat-sequence {
          tunnel: [w193] -> w180
          frame #0 {
            n93 = Wait (ms)(milliseconds to wait=u32 3000 ("等待时间（毫秒）")) -> ()  [unwired: 1 out]
          }
          frame #1 {
            n94 = local read "第一点校准值"() -> (w192:dbl)
            n95 = local read "第一点信号值"() -> (w190:dbl)
            n96 = local read "标液1"() -> (w189:sgl)
            n97 = Format Into String(format string="校准结果：\n校准值=%#.2f，信号值=%#.2f，标准值=%#.2f。" ("提示"), w192, w190, w189) -> (resulting string=w193:string)  [unwired: 2 in, 1 out]
          }
        }
        n98 = call "Add State to Queue.vi"("State(s) In (\"\")"="init: all\nCal: Over\nidle" ("State(s) In (\"\")")) -> ("States Out"=w177:string)  [unwired: 14 in]
        n99 = global read "多参数全局变量.vi" "多参数编号"() -> (w184:string)
        n100 = Format Into String(format string="编号：%s\n参数：%s\n信息：%s" ("格式字符串"), w184, w183, w180) -> (resulting string=w181:string)  [unwired: 2 in, 1 out]
        n101 = One Button Dialog(message=w181) -> ()  [unwired: 1 in, 1 out]
        n102 = call "校准日志.vi"("table"="校准记录", "日志信息"=w181) -> ()  [unwired: 9 in, 1 out]
      }
      frame "Cal: Over" {
        n103 = global read "多参数全局变量.vi" "校准运行状态"() -> (w195:T7)
        n104 = Bundle By Name(cluster=w195, "Cond"=FALSE) -> (w196:T7)
        n105 = global write "多参数全局变量.vi" "校准运行状态"(w196) -> ()
      }
      frame "idle", Default {
        n106 = event shown="[0] 超时" {
          selector: _ -> [_ _ _ _ _ _ _]
          dyn-events: _ -> [_ _ _ _ _ _ _]
          timeout: 10 -> [_ _ _ _ _ _ _]
          tunnel: w208 -> [w211 w215 w220 w226 w231 w243 _]
          tunnel: [w210 w214 w221 w230 w233 w242 w245] -> w207
          tunnel: [w209 w212 w222 w229 w232 w240 w246] -> w206
          tunnel: w205 -> [w209 w212 w222 w229 w232 w240 w246]
          tunnel: w201 -> [_ _ _ w224 _ _ _]
          event Timeout {
            n107 = event-data() -> ()  [unwired: 1 in, 3 out]
            n108 = call "Add State to Queue.vi"("State(s) In (\"\")"=w211) -> ("States Out"=w210:string)  [unwired: 14 in]
          }
          event "校准模式": Value Change {
            n109 = event-data() -> ()  [unwired: 1 in, 6 out]
            n110 = call "Add State to Queue.vi"("State(s) In (\"\")"=w215, "State(s) At Back (\"\")"="init: all\nidle" ("State(s) In (\"\")")) -> ("States Out"=w214:string)  [unwired: 13 in]
          }
          event "标液1", "滤波设定": Mouse Down {
            n111 = event-data() -> ("CtlRef"=w219:refnum<vi>)  [unwired: 1 in, 7 out]
            n112 = property class="DigNum (严格)"(reference=w219) -> (reference out=w216:refnum<vi>, "Value"=w217:sgl)  [unwired: 1 in, 1 out]
            n113 = call "数字键盘.vi"("OldNumber"=w217) -> ("NewNumber"=w218:dbl)  [unwired: 1 in]
            n114 = property class="DigNum (严格)"(reference=w216, "Val(Sgnl)"=w218) -> ()  [unwired: 1 in, 2 out]
            n115 = call "Add State to Queue.vi"("State(s) In (\"\")"=w220) -> ("States Out"=w221:string)  [unwired: 14 in]
          }
          event "标液1": Value Change {
            n116 = event-data() -> ("NewVal"=w227:sgl)  [unwired: 1 in, 5 out]
            n117 = global read "多参数全局变量.vi" "MB session in"() -> (w228:refnum<class "MB_Master.lvclass">)
            n118 = call "纳清电导率_第一点校准数据写入.vi"("数值"=w227, "MB session in"=w228) -> ("error out"=w225:errorcluster)  [unwired: 8 in, 1 out]
            n119 = Enqueue Element At Opposite End(queue=w224, element=T1."Cond" ("元素"), error in (no error)=w225) -> ()  [unwired: 1 in, 3 out]
            n120 = call "Add State to Queue.vi"("State(s) In (\"\")"=w226) -> ("States Out"=w230:string)  [unwired: 14 in]
          }
          event "滤波设定": Value Change {
            n121 = event-data() -> ()  [unwired: 1 in, 6 out]
            n122 = flat-sequence {
              frame #0 {
                n123 = global read "断电保存变量.vi" "滤波设置"() -> (w236:T5)
                n124 = local read "滤波设定"() -> (w234:sgl)
                n125 = Bundle By Name(cluster=w236, "Cond"=w234) -> (w235:T5)
                n126 = global write "断电保存变量.vi" "滤波设置"(w235) -> ()
              }
              frame #1 {
                n127 = call "配置文件保存.vi"() -> ()  [unwired: 12 in]
              }
            }
            n128 = call "Add State to Queue.vi"("State(s) In (\"\")"=w231) -> ("States Out"=w233:string)  [unwired: 14 in]
          }
          event "校准启动": Value Change {
            n129 = event-data() -> ()  [unwired: 1 in, 6 out]
            n130 = global read "多参数全局变量.vi" "校准运行状态"() -> (w238:T7)
            n131 = Bundle By Name(cluster=w238, "Cond"=TRUE) -> (w239:T7)
            n132 = global write "多参数全局变量.vi" "校准运行状态"(w239) -> ()
            n133 = call "Add State to Queue.vi"("State(s) In (\"\")"=w243, "State(s) At Back (\"\")"="init: all\nCal: Place standard solution\n Cal: Calibration process\nidle" ("State(s) In (\"\")")) -> ("States Out"=w242:string)  [unwired: 13 in]
          }
          event "校准停止": Value Change {
            n134 = event-data() -> ()  [unwired: 1 in, 6 out]
            n135 = call "Add State to Queue.vi"("State(s) In (\"\")"="init: all\nCal: Over\nidle" ("State(s) In (\"\")")) -> ("States Out"=w245:string)  [unwired: 14 in]
          }
        }
      }
    }
  }
